vi "Open ECA200.vi"() -> (0 "错误输出":errorcluster, 2 "仪器存在":bool, 3 "VISA资源名称输出":refnum<visa-resource-name>)   [LabVIEW 2020]
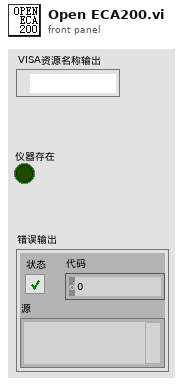
[diagram p1: front panel]
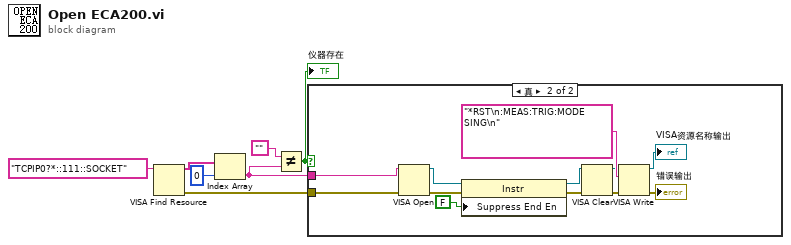
[diagram p0: block diagram]
diagram:
  n1 = VISA Find Resource(11:"TCPIP0?*::111::SOCKET" ("表达式(\"?*\")")) -> (0:w7:errorcluster, 3:w6:string[])  [unwired: 2 in, 1 out]
  n2 = Index Array(array=w6, index=0 ("索引")) -> (element=w3:string)
  n3 = Not Equal?(x="", y=w3) -> (x != y?=w1:bool)
  "仪器存在" <- w1
  n4 = case shown="真" w1 {
    tunnel: w7 -> [_ w19]
    tunnel: w3 -> [_ w18]
    frame False {
    }
    frame True {
      n5 = VISA Open(error in (no error)=w19, VISA resource name=w18) -> (VISA resource name=w16:refnum<visa-resource-name>, error out=w15:errorcluster)  [unwired: 3 in]
      n6 = property class="Instr"(reference=w16, error in=w15, "Suppress End En"=FALSE ("Message Based Settings:Suppress End Enable")) -> (reference out=w14:refnum<visa-resource-name>, error out=w13:errorcluster)
      n7 = VISA Clear(VISA resource name=w14, error in (no error)=w13) -> (VISA resource name out=w11:refnum<visa-resource-name>, error out=w10:errorcluster)
      n8 = VISA Write(VISA resource name=w11, write buffer="*RST\n:MEAS:TRIG:MODE SING\n" ("写入缓冲区"), error in (no error)=w10) -> (VISA resource name out=→"VISA资源名称输出":refnum<visa-resource-name>, error out=→"错误输出":errorcluster)  [unwired: 1 out]
    }
  }
